vi "formater commande si retour.vi"(1 "Tab cmde GPAO IN":string[][](array[string])=[["12-216C-04521", "EQIFIL ", "104mA    230ohm", "03104/08-05.01.01", "3", "221769", "EMAIL VOM 01.04.08  ", "BLATTY AG", "", "      ", "Fluid Automation Systems SA             ", "ALL", "0"], ["12-216C-04521", "EQIFIL ", "104mA    230ohm", "03128/08-01.01.01", "2", "226006", "RETURN FROM VIASYS2 ", "Fluid Automat. Systems GmbH", "", "      ", "Fluid Automation Systems SA             ", "ALL", "1"], ["12-216C-04521", "EQIFIL ", "104mA    230ohm", "03130/08-01.01.01", "1", "226005", "RETURN FROM VIASYS1 ", "Fluid Automat. Systems GmbH", "", "      ", "Fluid Automation Systems SA             ", "ALL", "1"], ["12-216C-04521", "EQIFIL ", "104mA    230ohm", "03365/08-01.01.01", "4", "225536", "SANS PAPIERS GE     ", "Fluid Automat. Systems GmbH", "", "      ", "Fluid Automation Systems SA             ", "ALL", "1"], ["12-216C-04521", "EQIFIL ", "104mA    230ohm", "03570/08-02.01.01", "100", "225052", "SANS PAPIERS        ", "IMI International Sp. z o.o.", "", "      ", "Fluid Automation Systems SA             ", "ANG", "1"], ["12-216C-04521", "EQIFIL ", "104mA    230ohm", "05066/08-01.01.01", "13", "225726", "120830              ", "Fluid Automat. Systems GmbH", "", "      ", "Fluid Automation Systems SA             ", "ALL", "1"], ["12-216C-04521", "EQIFIL ", "104mA    230ohm", "05067/08-01.01.01", "11", "225727", "120831              ", "Fluid Automat. Systems GmbH", "", "      ", "Fluid Automation Systems SA             ", "ALL", "1"]]) -> (0 "Tab cmde GPAO OUT":string[][](array[string])=[["12-216C-04521", "EQIFIL ", "104mA    230ohm", "03104/08-05.01.01", "3", "221769", "EMAIL VOM 01.04.08  ", "BLATTY AG", "", "      ", "Fluid Automation Systems SA             ", "ALL", "0"], ["12-216C-04521", "EQIFIL ", "104mA    230ohm", "03128/08-01.01.01", "2", "226006", "RETURN FROM VIASYS2 ", "Fluid Automat. Systems GmbH", "", "      ", "Fluid Automation Systems SA             ", "ALL", "1"], ["12-216C-04521", "EQIFIL ", "104mA    230ohm", "03130/08-01.01.01", "1", "226005", "RETURN FROM VIASYS1 ", "Fluid Automat. Systems GmbH", "", "      ", "Fluid Automation Systems SA             ", "ALL", "1"], ["12-216C-04521", "EQIFIL ", "104mA    230ohm", "03365/08-01.01.01", "4", "225536", "SANS PAPIERS GE     ", "Fluid Automat. Systems GmbH", "", "      ", "Fluid Automation Systems SA             ", "ALL", "1"], ["12-216C-04521", "EQIFIL ", "104mA    230ohm", "03570/08-02.01.01", "100", "225052", "SANS PAPIERS        ", "IMI International Sp. z o.o.", "", "      ", "Fluid Automation Systems SA             ", "ANG", "1"], ["12-216C-04521", "EQIFIL ", "104mA    230ohm", "05066/08-01.01.01", "13", "225726", "120830              ", "Fluid Automat. Systems GmbH", "", "      ", "Fluid Automation Systems SA             ", "ALL", "1"], ["12-216C-04521", "EQIFIL ", "104mA    230ohm", "05067/08-01.01.01", "11", "225727", "120831              ", "Fluid Automat. Systems GmbH", "", "      ", "Fluid Automation Systems SA             ", "ALL", "1"]])   [LabVIEW 2020]
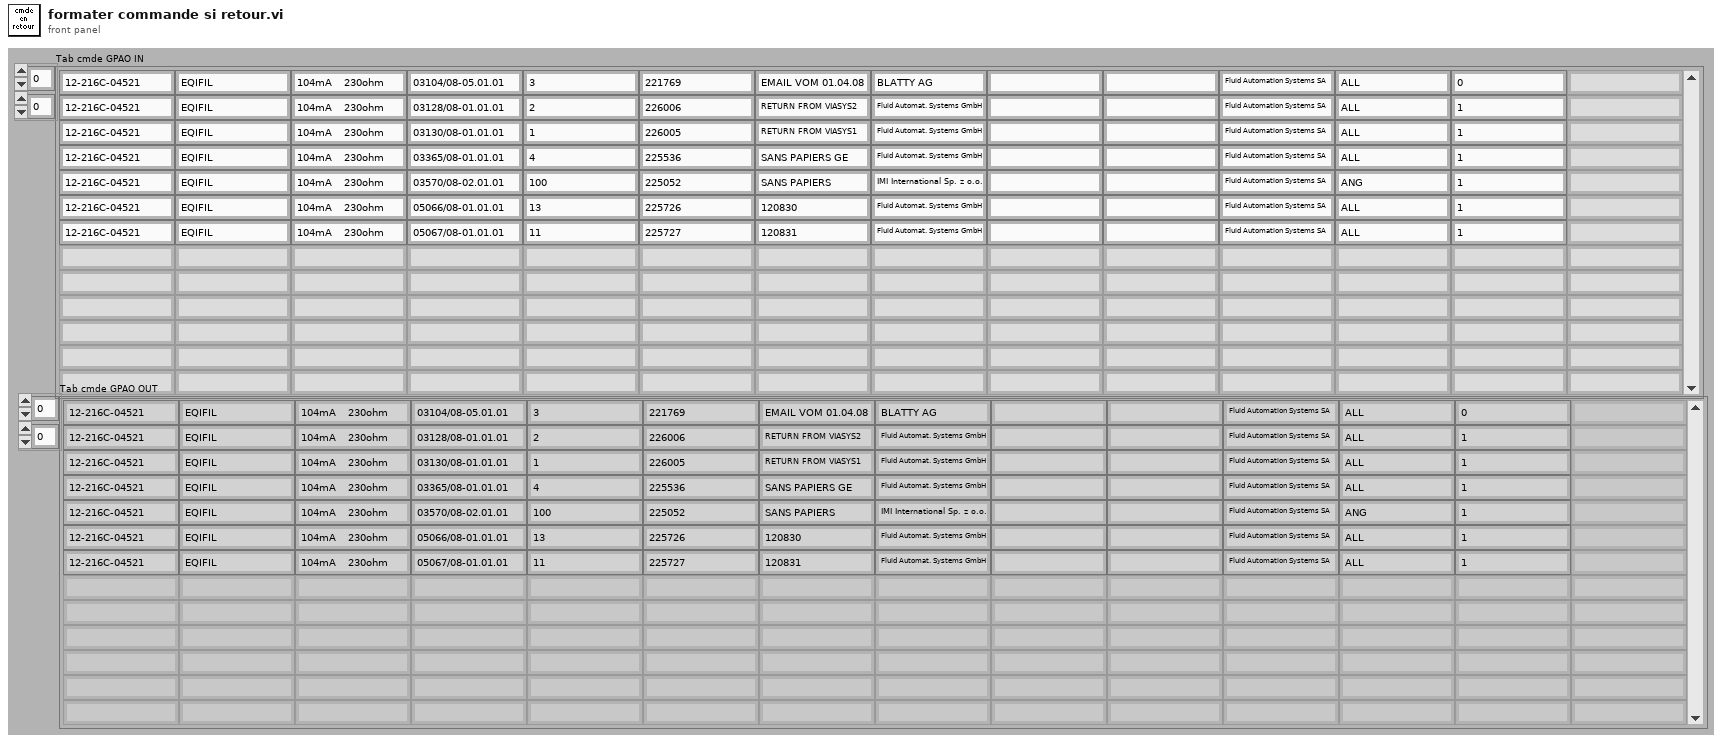
[diagram p1: front panel]
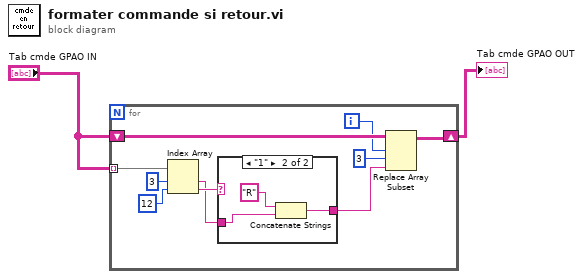
[diagram p0: block diagram]
diagram:
  n1 = for {
    tunnel: "Tab cmde GPAO IN" -> [w12] mode=indexing
    shift-right: [w6] -> w1
    shift-left: "Tab cmde GPAO IN" -> [w7]
    i -> [w5]
    n2 = Index Array(array=w12, index #1=3 ("indice"), index #2=12 ("indice")) -> (element #1=w8:string, element #2=w9:string)
    n3 = case shown="\"1\"" w9 {
      tunnel: w8 -> [w13 w15]
      tunnel: [w13 w14] -> w3
      frame "0", Default {
      }
      frame "1" {
        n4 = Concatenate Strings("R", w15) -> (w14:string)
      }
    }
    n5 = Replace Array Subset(array=w7, new element=w3, index (row)=w5, index (col)=3 ("indice désactivé (col)")) -> (w6:string[][])
  }
  "Tab cmde GPAO OUT" <- w1
